vi "append_h5_dataset.vi"(8 "error in (no error)":errorcluster, 9 "Data":sgl[](array[numeric]), 11 "dset in":T1 format="%.0x") -> (0 "error out":errorcluster)   [LabVIEW 2015]
uses:
  <vilib>/addons/h5labview2/base/hid_t.ctl
  <vilib>/addons/h5labview2/base/lib_path.vi
  <vilib>/addons/h5labview2/base/H5Equery.vi
  <vilib>/addons/h5labview2/dataset/H5Dwrite.llb/H5Dwrite.xnode
  <vilib>/addons/h5labview2/dataset/H5D.lvlib
  <vilib>/addons/h5labview2/space/H5S.lvlib
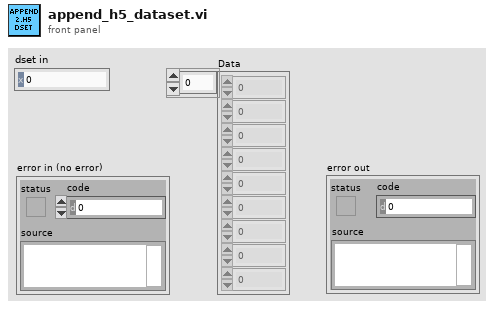
[diagram p1: front panel]
types:
  T1 = typedef "hid_t.ctl" = i32
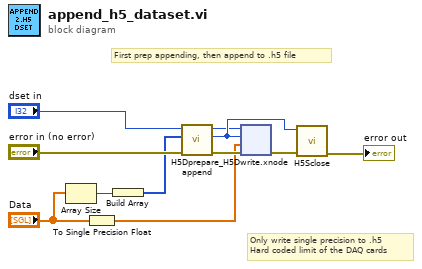
[diagram p0: block diagram]
diagram:
  # "First prep appending, then append to .h5 file"
  # "Only write single precision to .h5 \nHard coded limit of the DAQ cards"
  n1 = Array Size(array="Data") -> (size(s)=w2:i32)
  n2 = To Single Precision Float(number="Data") -> (single precision float=w3:sgl[])
  n3 = Build Array(w2) -> (w4:i32[])
  n4 = call <vilib>:"H5Dprepare_append.vi"("error in (no error)"="error in (no error)", "append dims"=w4, "dset in"="dset in") -> ("error out"=w10:errorcluster, "space out"=w11:T1, "dset out"=w9:T1)  [unwired: 6 in]
  n5 = xnode "H5Dwrite.xnode"("error in (no error)"=w10, "data"=w3, "file space"=w11, "ref in"=w9) -> ("error out"=w8:errorcluster)  [unwired: 3 in, 2 out]
  n6 = call <vilib>:"H5Sclose.vi"("error in (no error)"=w8, "space in"=w11) -> ("error out"=→"error out":errorcluster)  [unwired: 9 in]
